vi "deviceAnalysisTest_3Tach_DigitalTach.vi"() -> ()   [LabVIEW 2017]
uses:
  <vilib>/addons/InsightCM/MessageBus/Base/KeyValuePairs.ctl
  <vilib>/addons/InsightCM/MessageBus/Base/controls/AlarmRuleEntry.ctl
  <vilib>/addons/InsightCM/Devices/Shared/DataAccessors/controls/channelType_StatusLookup.ctl
  <vilib>/addons/InsightCM/MessageBus/Base/ConfigurableMetric.ctl
  <vilib>/addons/InsightCM/Utilities/ChannelStatus/controls/status.ctl
  <vilib>/addons/InsightCM/Utilities/ChannelStatus/controls/statusState.ctl
  <vilib>/addons/InsightCM/Devices/Shared/ConfigurationParsing/controls/filePaths.ctl
panel:
  out "FeatureLookup":variant
  in  "milliseconds to wait":u32=100
  in  "Tab Control":T1(tab)
  in  "Root Directory":path=path "C:/Users/Administrator/Desktop/testDevice files/speedProfile"
  in  "Configuration Files":T2={"AlarmRules"=path "AlarmRules.json", "MetricCfg"=path "MetricConfigs.json", "HierarchyNode"=path "Hierarchy.json", "DeviceModel"=path "DeviceModel.json"}
  in  "sampling info":cluster{"Fs":dbl, "#s":dbl}={"Fs"=10000.0, "#s"=10000.0} {"Fs" format="%.2p"}
  in  "Vibration 3":T3(array[cluster])
  in  "Tachometer 3":cluster{"RPM":sgl}={"RPM"=60.0} {"RPM" scale=1.0..6000.0}
  in  "Vibration 2":T3(array[cluster])
  in  "Tachometer 2":cluster{"RPM":sgl}={"RPM"=60.0} {"RPM" scale=1.0..6000.0}
  in  "Vibration":T3(array[cluster])
  in  "Tachometer":cluster{"RPM":sgl}={"RPM"=60.0} {"RPM" scale=1.0..6000.0}
  out "Waveform Graph":waveform(dbl)[](graph)
  out "Waveform Graph 2":waveform(sgl)[](graph)
  in  "stop":bool
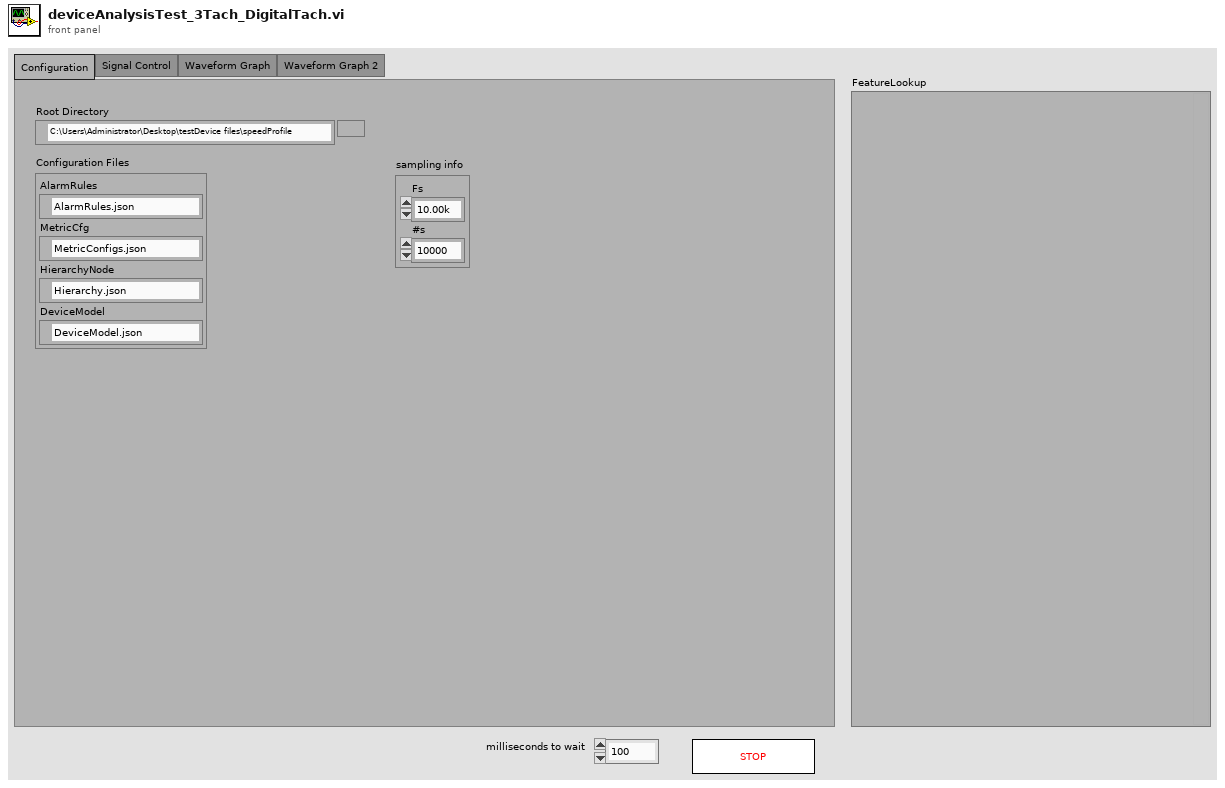
[diagram p1: front panel]
types:
  T1 = enum32{"Configuration", "Signal Control", "Waveform Graph", "Waveform Graph 2"}
  T2 = typedef "ConfigurationParsing.lvlib/filePaths.ctl" = cluster{"AlarmRules":path, "MetricCfg":path, "HierarchyNode":path, "DeviceModel":path}
  T3 = cluster{"order.":dbl, "mag (rms)":dbl, "phase (°)":dbl}[][]
  T4 = typedef "ChannelStatus.lvlib/statusState.ctl" = cluster{"channelAlias":string, "current":T5, "previous":T5, "changed":bool}
  T5 = typedef "ChannelStatus.lvlib/status.ctl" = enum16{"init", "ok", "open", "short", "outOfRange"}
  T6 = typedef "ConfigurableMetric.ctl" = cluster{"Id":i32, "MetricType":string, "Name":string, "Locked":bool, "Properties":T7}
  T7 = typedef "KeyValuePairs.ctl" = cluster{"Key":string, "Value":string}[]
  T8 = cluster{"order.":dbl, "mag (rms)":dbl, "phase (°)":dbl}[]
  T9 = typedef "AlarmRuleEntry.ctl" = cluster{"Id":i32, "State":string, "Path":string, "Message":string, "DeviceOnly":bool, "Configuration":cluster{"Condition":string, "SetPoint":string, "Type":string, "Hysteresis":dbl, "OnDelaySeconds":dbl, "OffDelaySeconds":dbl}, "Severity":i32}
  T10 = typedef "ConfigurationParsing.lvlib/DeviceConfigData.ctl" = cluster{"Device Info":T11, "AcquisitionProperties":variant, "Channels":variant[], "StreamingProperties":variant, "DeviceSystemProperties":variant}
  T11 = typedef "ConfigurationParsing.lvlib/deviceInfo.ctl" = cluster{"Config Version":string, "DeviceID":string}
  T12 = typedef "DeviceModel.ctl" = cluster{"AssetModel":T13, "SoftwareModel":T14}
  T13 = typedef "AssetModel.ctl" = cluster{"Id":i32, "PhysicalName":string, "LogicalName":string, "PluginCodename":string, "FirmwareInfo":string, "HardwareConfig":string, "SoftwareConfigId":i32, "HierarchyNodeId":i32}
  T14 = typedef "SoftwareModel.ctl" = cluster{"Id":i32, "DeviceAssetModelId":i32, "Version":string, "Config":string, "DeviceProperties":T7, "Channels":T15[]}
  T15 = typedef "BlueRidgeChannel.ctl" = cluster{"Id":i32, "ChannelId":string, "Name":string, "ChannelCategory":string, "ChannelType":string, "ChannelTypeList":string, "HierarchyNodeId":i32, "Enabled":bool, "Properties":T7, "MetricConfigurations":T16[]}
  T16 = typedef "MetricConfiguration.ctl" = cluster{"Id":i32, "ChannelCategory":string, "MeasurementType":string, "Metrics":T17[]}
  T17 = typedef "MetricInstance.ctl" = cluster{"Id":i32, "Codename":string, "DisplayName":string, "Unit":string, "Unscaled":bool, "Locked":bool, "TagPath":string, "Properties":T7}
  T18 = cluster{"AlarmRules":variant, "MetricCfg":variant, "HierarchyNode":variant, "DeviceConfig":T10, "DeviceModel":T12}
  T19 = typedef "AnalysisDevice.ctl" = cluster{"Device Id":string, "Dynamic Channels":T20[], "Static Channels":T28[]}
  T20 = typedef "AnalysisDynamicChannel.ctl" = cluster{"ChannelName":string, "Sensor Type":T21, "Conversion Op":T22, "Features":T23[], "Data":waveform(sgl), "Speed":sgl, "SP Index":i32, "Properties":variant, "Data Valid":bool, "Calc Measurement Type":T27}
  T21 = typedef "AnalysisSensorType.ctl" = enum16{"Accelerometer", "Velocity", "Displacement", "Tachometer", "Tempertature ", "dynamicVoltage", "Voltage", "Current", "Microphone", "Resistance", "Digital Input", "<Unknown>"}
  T22 = typedef "AnalysisConversionOp.ctl" = enum16{"none", "singleInt", "doubleInt", "singleDiff", "doubleDiff"}
  T23 = typedef "AnalysisFeature.ctl" = cluster{"Type":i32, "Code Name":string, "Unit":string, "Display Name":string, "Value":sgl, "Start":dbl, "Stop":dbl, "Band Domain":T24, "Band Calc":T25, "Amplitude Scale":T26, "Tag Path":string, "Conversion Op (phase sb only)":T22, "sbp code letter":string}
  T24 = typedef "AnalysisBandDomain.ctl" = enum16{"Frequency", "CPM", "Orders"}
  T25 = typedef "AnalysisBandCalculation.ctl" = enum16{"Total", "Max", "Phase"}
  T26 = typedef "AnalysisBandAmplitudeScale.ctl" = enum16{"rms", "peak", "pk-pk", "phase", "<none>"}
  T27 = typedef "AnalysisCalculatedMeasurementType.ctl" = enum16{"acceleration", "velocity", "displacement", "tachometer", "speed", "temperature", "voltage", "current", "resistance", "digitalInput", "<Unknown>"}
  T28 = typedef "AnalysisStaticChannel.ctl" = cluster{"ChannelName":string, "Sensor Type":T21, "Features":T23[], "Properties":variant, "Data Valid":bool, "Calc Measurement Type":T27, "Acquisition Timestamp":timestamp}
  T29 = typedef "AnalysisState.ctl" = cluster{"Properties":cluster{"File Properties":variant, "Static Properties":variant, "Waveform Properties":variant}, "Properties Initialized?":bool, "Device":T19, "Speed Profiles":T30[]}
  T30 = typedef "AnalysisSpeedProfile.ctl" = cluster{"t0":dbl, "pulse positions":sgl[], "speed":dbl}
  T31 = typedef "AnalysisBOP.lvlib/AnalysisGroups.ctl" = cluster{"StaticChannels":T32[], "TachVibrationGroups":T34[]}
  T32 = typedef "AnalysisBOP.lvlib/GeneralStaticChanAnalysisCfg.ctl" = cluster{"Wfm Index":i32, "ChannelName":string, "ChannelID":string, "bounds":T33, "TagPath":string, "Triggerable":bool}
  T33 = typedef "ChannelStatus.lvlib/outOfRangeBounds.ctl" = cluster{"maximum":dbl, "minimum":dbl}
  T34 = typedef "AnalysisBOP.lvlib/TachVibrationGroupCfg.ctl" = cluster{"TachometerChanAnalysisConfig":T35, "AnalysisChannels":T36[]}
  T35 = typedef "AnalysisBOP.lvlib/TachometerChanAnalysisCfg.ctl" = cluster{"Wfm Index":i32, "ChannelName":string, "ChannelID":string, "PulsesPerRevolution":sgl, "TachometerThreshold":sgl, "TachometerSlope":string, "TachometerHysteresis":sgl, "sampleRate":dbl, "tachometerType":string, "Analysis Wfm Index":i32}
  T36 = typedef "AnalysisBOP.lvlib/VibrationChanAnalysisCfg.ctl" = cluster{"Wfm Index":i32, "ChannelName":string, "ChannelID":string, "speedRatio":dbl, "MeasurementType":string}
  T37 = typedef "channelType_StatusLookup.ctl" = enum16{"Static", "Dynamic"}
  T38 = typedef "rolloverState.ctl" = cluster{"prev value":u32, "total add":dbl}
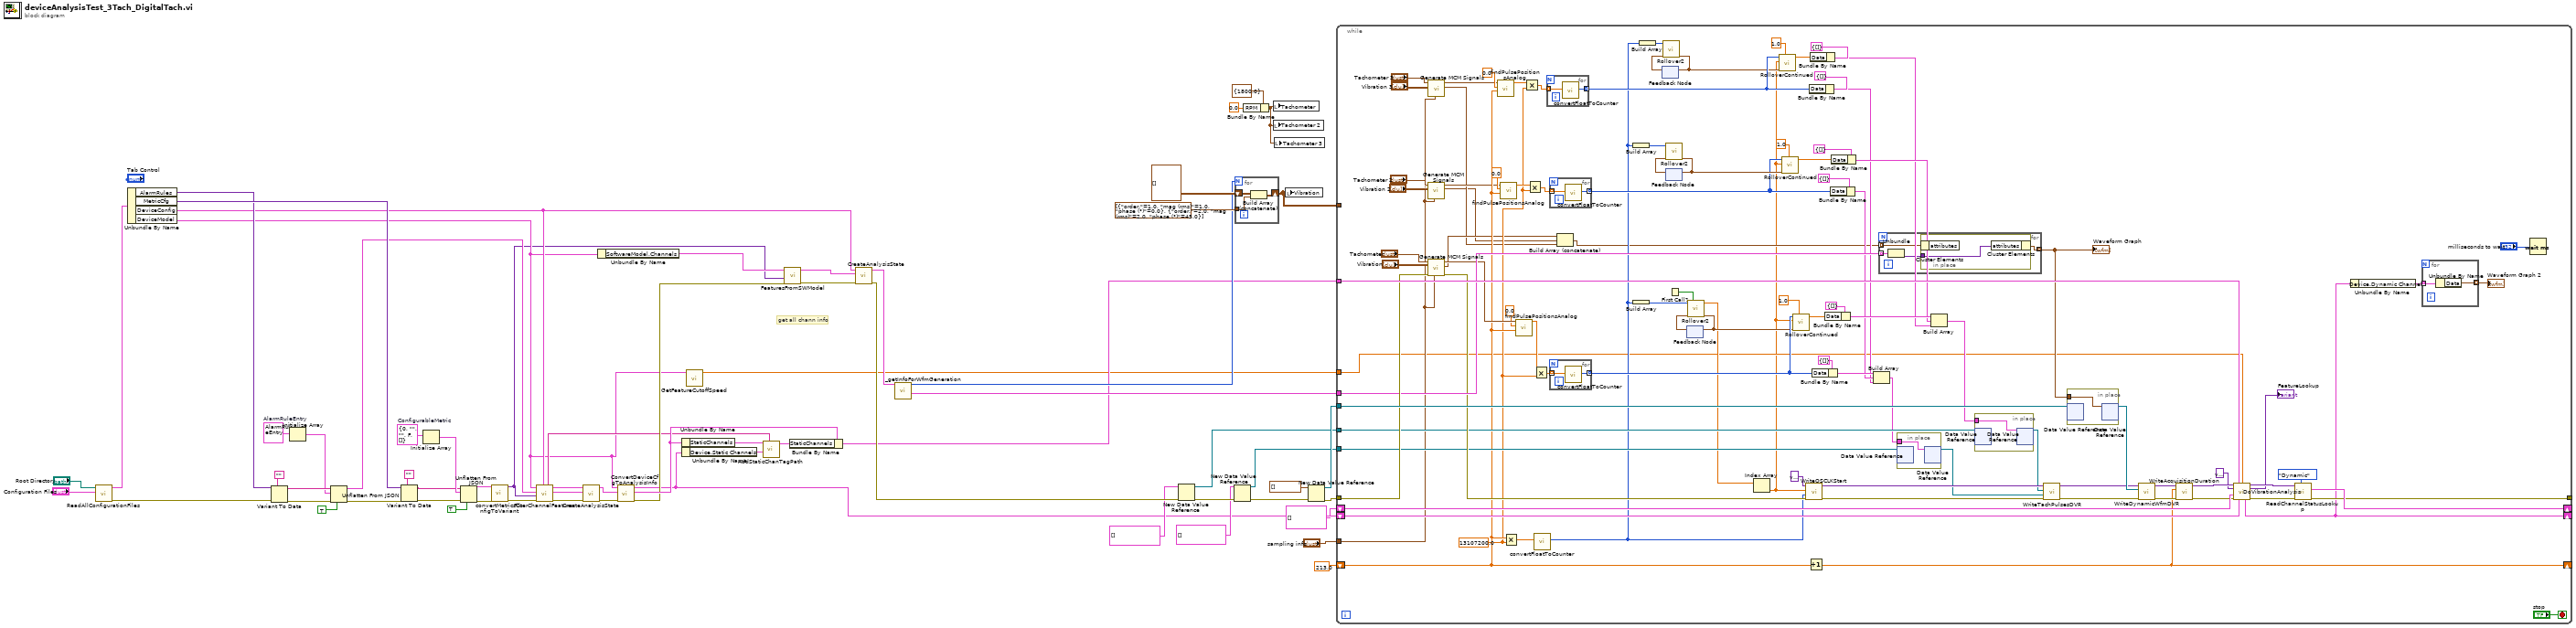
[diagram p0: block diagram]
diagram:
  w20 = T6 {"Id"=0, "MetricType"="", "Name"="", "Locked"=FALSE, "Properties"=[]}  # ConfigurableMetric
  w49 = T9 {"Id"=0, "State"="", "Path"="", "Message"="", "DeviceOnly"=FALSE, "Configuration"={"Condition"="", "SetPoint"="", "Type"="", "Hysteresis"=0.0, "OnDelaySeconds"=0.0, "OffDelaySeconds"=0.0}, "Severity"=0}  # AlarmRuleEntry
  # "get all chann info"
  n1 = call <vilib>:"ReadAllConfigurationFiles.vi"("Configuration Files"="Configuration Files", "Root Directory"="Root Directory") -> ("error out"=w12:errorcluster, "Configuration"=w61:T18)  [unwired: 6 in, 2 out]
  n2 = Unbundle By Name(w61) -> ("AlarmRules"=w46:variant, "MetricCfg"=w55:variant, "DeviceConfig"=w30:T10, "DeviceModel"=w5:T12)
  n3 = Variant To Data(error in=w12, type="", Variant=w46) -> (data=w50:string, error out=w52:errorcluster)
  n4 = Initialize Array(w49) -> (w48:T9[])  [unwired: 1 in]
  n5 = Unflatten From JSON(JSON string=w50, type and defaults=w48, default null elements? (F)=TRUE, error in (no error)=w52) -> (value=w31:T9[], error out=w47:errorcluster)  [unwired: 3 in]
  n6 = Variant To Data(error in=w47, type="", Variant=w55) -> (data=w56:string, error out=w59:errorcluster)
  n7 = Initialize Array(w20) -> (w57:T6[])  [unwired: 1 in]
  n8 = Unflatten From JSON(JSON string=w56, type and defaults=w57, default null elements? (F)=TRUE, error in (no error)=w59) -> (value=w54:T6[], error out=w45:errorcluster)  [unwired: 3 in]
  n9 = call <vilib>:"convertMetricsConfigToVariant.vi"("error in (no error)"=w45, "MetricInstanceConfigs"=w54) -> ("error out"=w62:errorcluster, "metricInstanceConfig"=w1:variant)  [unwired: 8 in]
  n10 = call <vilib>:"FilterChannelFeatures.vi"("DeviceConfig"=w30, "error in (no error)"=w62, "Metric Lookup"=w1, "AlarmRules"=w31, "DeviceModel"=w5) -> ("error out"=w65:errorcluster, "Device"=w63:T19, "DeviceConfig Out"=w64:T10, "trigger list"=w6:string[])  [unwired: 3 in]
  n11 = call <vilib>:"CreateAnalysisState.vi"("error in (no error)"=w65, "Device"=w63, "DeviceConfig"=w64) -> ("error out"=w11:errorcluster, "Analysis State"=w9:T29)  [unwired: 7 in]
  n12 = Unbundle By Name(w5) -> ("SoftwareModel.Channels"=w21:T15[])
  n13 = call <vilib>:"ConvertDeviceCfgToAnalysisInfo.vi"("error in (no error)"=w11, "Analysis State"=w9, "DeviceModel"=w5) -> ("error out"=w10:errorcluster, "AnalysisGroups"=w13:T31, "Analysis State out"=w8:T29)  [unwired: 5 in, 1 out]
  n14 = Unbundle By Name(w13) -> ("StaticChannels"=w16:T32[])
  n15 = Unbundle By Name(w8) -> ("Device.Static Channels"=w17:T28[])
  n16 = call <vilib>:"GetFeatureCutoffSpeed.vi"("DeviceModel"=w5) -> ("featureCutoffSpeed"=w4:dbl)  [unwired: 10 in]
  n17 = call <vilib>:"AddStaticChanTagPath.vi"("trigger list"=w6, "Device.Static Channels"=w17, "StaticChannels"=w16) -> ("StaticChannels out"=w15:T32[])  [unwired: 8 in]
  n18 = call <vilib>:"FeaturesFromSWModel.vi"("error in (no error)"=w10, "Band Cache"=w1, "Channels"=w21) -> ("error out"=w3:errorcluster, "Device"=w2:T19)  [unwired: 7 in]
  n19 = Bundle By Name(cluster=w13, "StaticChannels"=w15) -> (w14:T31)
  n20 = call <vilib>:"CreateAnalysisState.vi"("error in (no error)"=w3, "Device"=w2, "DeviceConfig"=w30) -> ("error out"=w27:errorcluster, "Analysis State"=w32:T29)  [unwired: 7 in]
  n21 = call <vilib>:"_getInfoForWfmGeneration.vi"("Analysis State"=w32) -> ("wfm info"=w33:cluster{i32, "variant":variant}[], "number of channels"=w34:i32)  [unwired: 9 in]
  n22 = New Data Value Reference(data value=cluster{"Data":dbl[]}[] [] ("Keyphasor Pulses"), error in=w27) -> (data value reference=w23:refnum<data-value>, error out=w28:errorcluster)
  n23 = New Data Value Reference(data value=cluster{"Data":u32[]}[] [] ("Keyphasor Pulses U32"), error in=w28) -> (data value reference=w24:refnum<data-value>, error out=w29:errorcluster)
  n24 = for {
    N: w34 -> [_]
    tunnel: T8 [{"order."=1.0, "mag (rms)"=1.0, "phase (°)"=0.0}, {"order."=2.0, "mag (rms)"=2.0, "phase (°)"=45.0}] ("Vibration") -> [w68]
    shift-right: [w67] -> w37
    shift-left: T3 [] -> [w66]
    n25 = Build Array (concatenate)(w66, w68) -> (w67:T3)
  }
  n26 = Bundle By Name(cluster=cluster{"RPM":sgl} {"RPM"=1800.0} ("Tachometer"), "RPM"=sgl 0.0) -> (w19:cluster{"RPM":sgl})
  n27 = local write "Tachometer"(w19) -> ()
  n28 = local write "Tachometer 2"(w19) -> ()
  n29 = local write "Tachometer 3"(w19) -> ()
  n30 = local write "Vibration"(w37) -> ()
  n31 = New Data Value Reference(data value=waveform(sgl)[] [] ("wfmData"), error in=w29) -> (data value reference=w41:refnum<data-value>, error out=w42:errorcluster)
  n32 = while {
    tunnel: w42 -> [w155]
    tunnel: w14 -> [w166]
    shift-right: [w165] -> _
    shift-left: T4[] [] ("channel status") -> [w164]
    tunnel: w41 -> [w159]
    tunnel: "sampling info" -> [w107]
    tunnel: w37 -> [_]
    tunnel: [w148] -> _
    tunnel: w33 -> [w147]
    shift-right: [w144] -> _
    shift-left: w8 -> [w145]
    tunnel: w24 -> [w134]
    tunnel: w23 -> [w135]
    shift-right: [w125] -> _
    shift-left: 213.0 -> [w84]
    tunnel: w4 -> [w73]
    stop <- "stop" stop-if-true
    w83 = 13107200.0
    n33 = call <vilib>:"Generate MCM Signals.vi"("sampling info"=w107, "Vibration"="Vibration 2", "Tachometer"="Tachometer 2") -> ("Vibration signals"=w74:waveform(dbl)[], "Tach signal"=w78:waveform(dbl))  [unwired: 6 in, 1 out]
    n34 = call <vilib>:"Generate MCM Signals.vi"("sampling info"=w107, "error in"=w155, "Vibration"="Vibration", "Tachometer"="Tachometer") -> ("error out"=w136:errorcluster, "Vibration signals"=w79:waveform(dbl)[], "Tach signal"=w130:waveform(dbl))  [unwired: 5 in]
    n35 = call <vilib>:"Generate MCM Signals.vi"("sampling info"=w107, "Vibration"="Vibration 3", "Tachometer"="Tachometer 3") -> ("Vibration signals"=w75:waveform(dbl)[], "Tach signal"=w76:waveform(dbl))  [unwired: 6 in, 1 out]
    n36 = call <vilib>:"findPulsePositionsAnalog.vi"("t0"=w84, "Level"=0.0, "Tach signal"=w76) -> ("pulse positions"=w86:dbl[])  [unwired: 8 in]
    n37 = call <vilib>:"findPulsePositionsAnalog.vi"("t0"=w84, "Level"=0.0, "Tach signal"=w78) -> ("pulse positions"=w105:dbl[])  [unwired: 8 in]
    n38 = Multiply(x=w84, y=w83) -> (x*y=w119:dbl)
    n39 = call <vilib>:"findPulsePositionsAnalog.vi"("t0"=w84, "Level"=0.0, "Tach signal"=w130) -> ("pulse positions"=w124:dbl[])  [unwired: 8 in]
    n40 = Multiply(x=w86, y=w83) -> (x*y=w85:dbl[])
    n41 = Multiply(x=w105, y=w83) -> (x*y=w106:dbl[])
    n42 = Multiply(x=w124, y=w83) -> (x*y=w120:dbl[])
    n43 = call <vilib>:"convertFloatToCounter.vi"("Numeric"=w119) -> ("Counter Version"=w82:u32)  [unwired: 10 in]
    n44 = for {
      tunnel: w85 -> [w168] mode=indexing
      tunnel: [w167] -> w92 mode=indexing
      n45 = call <vilib>:"convertFloatToCounter.vi"("Numeric"=w168) -> ("Counter Version"=w167:u32)  [unwired: 10 in]
    }
    n46 = for {
      tunnel: w106 -> [w170] mode=indexing
      tunnel: [w169] -> w98 mode=indexing
      n47 = call <vilib>:"convertFloatToCounter.vi"("Numeric"=w170) -> ("Counter Version"=w169:u32)  [unwired: 10 in]
    }
    n48 = for {
      tunnel: w120 -> [w172] mode=indexing
      tunnel: [w171] -> w115 mode=indexing
      n49 = call <vilib>:"convertFloatToCounter.vi"("Numeric"=w172) -> ("Counter Version"=w171:u32)  [unwired: 10 in]
    }
    n50 = Build Array (concatenate)(w79, w74, w75) -> (w77:waveform(dbl)[])
    n51 = Build Array(w82) -> (w100:u32[])
    n52 = Build Array(w82) -> (w116:u32[])
    n53 = Build Array(w82) -> (w90:u32[])
    n54 = feedback #1() -> (w91:T38)  [unwired: 1 in]
    n55 = call <vilib>:"Rollover2.vi"("rollover state"=w91, "counter"=w90) -> ("rollover state"=w89:T38)  [unwired: 8 in, 1 out]
    n56 = feedback-in #1(w89) -> ()
    n57 = feedback #2() -> (w99:T38)  [unwired: 1 in]
    n58 = call <vilib>:"Rollover2.vi"("rollover state"=w99, "counter"=w100) -> ("rollover state"=w101:T38)  [unwired: 8 in, 1 out]
    n59 = feedback-in #2(w101) -> ()
    n60 = First Call?() -> (First Call?: T/F=w118:bool)
    n61 = feedback #3() -> (w117:T38)  [unwired: 1 in]
    n62 = call <vilib>:"Rollover2.vi"("reset"=w118, "rollover state"=w117, "counter"=w116) -> ("rollover state"=w114:T38, "counter"=w113:dbl[])  [unwired: 7 in]
    n63 = feedback-in #3(w114) -> ()
    n64 = Index Array(array=w113) -> (element=w71:dbl)  [unwired: 1 in]
    n65 = call <vilib>:"RolloverContinued.vi"("acq block size (s)"=1.0, "rollover state"=w89, "OSClkStart"=w71, "counter"=w92) -> ("this block"=w94:dbl[])  [unwired: 4 in, 3 out]
    n66 = call <vilib>:"RolloverContinued.vi"("acq block size (s)"=1.0, "rollover state"=w101, "OSClkStart"=w71, "counter"=w98) -> ("this block"=w96:dbl[])  [unwired: 4 in, 3 out]
    n67 = call <vilib>:"RolloverContinued.vi"("acq block size (s)"=1.0, "rollover state"=w114, "OSClkStart"=w71, "counter"=w115) -> ("this block"=w112:dbl[])  [unwired: 4 in, 3 out]
    n68 = call <vilib>:"WriteOSCLKStart.vi"("error in (no error)"=w136, "osclkStart U32"=w82, "osclkStart"=w71, "variant"=variant) -> ("error out"=w139:errorcluster, "variant"=w140:variant)  [unwired: 6 in]
    n69 = Increment(x=w84) -> (x+1=w125:dbl)
    n70 = Bundle By Name(cluster=cluster{"Data":u32[]} {"Data"=[]} ("PulsePositions"), "Data"=w92) -> (w81:cluster{"Data":u32[]})
    n71 = Bundle By Name(cluster=cluster{"Data":dbl[]} {"Data"=[]} ("PulsePositions"), "Data"=w94) -> (w80:cluster{"Data":dbl[]})
    n72 = Bundle By Name(cluster=cluster{"Data":u32[]} {"Data"=[]} ("PulsePositions"), "Data"=w115) -> (w123:cluster{"Data":u32[]})
    n73 = Bundle By Name(cluster=cluster{"Data":dbl[]} {"Data"=[]} ("PulsePositions"), "Data"=w112) -> (w127:cluster{"Data":dbl[]})
    n74 = Bundle By Name(cluster=cluster{"Data":u32[]} {"Data"=[]} ("PulsePositions"), "Data"=w98) -> (w102:cluster{"Data":u32[]})
    n75 = Bundle By Name(cluster=cluster{"Data":dbl[]} {"Data"=[]} ("PulsePositions"), "Data"=w96) -> (w95:cluster{"Data":dbl[]})
    n76 = Build Array(w123, w102, w81) -> (w121:cluster{"Data":u32[]}[])
    n77 = for {
      tunnel: w77 -> [w179] mode=indexing
      tunnel: w147 -> [w180] mode=indexing
      tunnel: [w178] -> w146 mode=indexing
      n78 = Unbundle(w180) -> ("variant"=w177:variant)  [unwired: 1 out]
      n79 = in-place {
        in-place-border: w177 -> [w181]
        n80 = in-place-cluster #4(w179) -> ()  [unwired: 1 out]
        n81 = in-place-cluster #4("attributes"=w181) -> (w178:waveform(dbl))
      }
    }
    "Waveform Graph" <- w146
    n82 = in-place {
      in-place-border: w121 -> [w173]
      n83 = in-place-dvr #5(w134) -> ()  [unwired: 2 out]
      n84 = in-place-dvr #5(w173) -> (w133:refnum<data-value>)  [unwired: 1 out]
    }
    n85 = Build Array(w127, w95, w80) -> (w126:cluster{"Data":dbl[]}[])
    n86 = in-place {
      in-place-border: w126 -> [w174]
      n87 = in-place-dvr #6(w135) -> ()  [unwired: 2 out]
      n88 = in-place-dvr #6(w174) -> (w132:refnum<data-value>)  [unwired: 1 out]
    }
    n89 = call <vilib>:"WriteTachPulsesDVR.vi"("error in (no error)"=w139, "tachometer pulses U32"=w133, "tachometerPulsesDVR"=w132, "variant"=w140) -> ("error out"=w138:errorcluster, "variant"=w131:variant)  [unwired: 6 in]
    n90 = in-place {
      in-place-border: w146 -> [w182]
      n91 = in-place-dvr #7(w159) -> ()  [unwired: 2 out]
      n92 = in-place-dvr #7(w182) -> (w158:refnum<data-value>)  [unwired: 1 out]
    }
    n93 = call <vilib>:"WriteDynamicWfmDVR.vi"("error in (no error)"=w138, "dynamic Wfm DVR"=w158, "variant"=w131) -> ("error out"=w163:errorcluster, "variant"=w162:variant)  [unwired: 7 in]
    n94 = call <vilib>:"WriteAcquisitionDuration.vi"("error in (no error)"=w163, "acquisitionDuration"=w125, "variant"=w162) -> ("error out"=w160:errorcluster, "variant"=w161:variant)  [unwired: 7 in]
    n95 = call <vilib>:"DoVibrationAnalysis.vi"("variant"=w161, "AnalysisGroups"=w166, "FeatureSpeedCutoff"=w73, "featureLookup"=variant, "channel status"=w164, "error in (no error)"=w160, "Analysis State"=w145) -> ("variant out"=w151:variant, "FeatureLookup"=→"FeatureLookup":variant, "Analysis State Out"=w144:T29, "error out"=w150:errorcluster)  [unwired: 4 in, 1 out]
    n96 = call <vilib>:"ReadChannelStatusLookup.vi"("channel type"=channelType_StatusLookup."Dynamic", "error in (no error)"=w150, "variant"=w151) -> ("error out"=w148:errorcluster, "channel status"=w165:T4[])  [unwired: 6 in, 1 out]
    n97 = Unbundle By Name(w144) -> ("Device.Dynamic Channels"=w143:T20[])
    n98 = for {
      tunnel: w143 -> [w176] mode=indexing
      tunnel: [w175] -> w142 mode=indexing
      n99 = Unbundle By Name(w176) -> ("Data"=w175:waveform(sgl))
    }
    "Waveform Graph 2" <- w142
    n100 = Wait (ms)(milliseconds to wait="milliseconds to wait") -> ()  [unwired: 1 out]
  }
